vi "Keithley 182 Reading Config.VI"(1 "User Relative Value":dbl min=-30.3 max=30.3 format="%.9f", 2 "Reading Source":u16(ring) items=["Latest Reading from A/D", "One Reading from buffer", "All Readings in buffer", "Maximum Value in buffer", "Mimimum Value in buffer"], 4 "error in":T1, 5 "Analog Output Relative":u16(ring) items=["Disable Reading Relative", "Enable Reading Relative using current reading", "Enable Reading Relative using Value", "Enable Reading Relative, use present value"], 6 "Reading Format":u16(ring), 7 "VISA resource name":refnum<visa-resource-name>) -> (0 "error out":T1, 3 "VISA resource name out":refnum<visa-resource-name>)   [LabVIEW 2015]
doc: "This VI allows you to configure the 182 Reading source, format, and reading relative.\nOptions:\n\nReading Source\n0 = Latest Reading from A/D converter\n1 = One reading from buffer\n2 = All readings in buffer\n3 = Maximum value in buffer\n4 = Minimum value in buffer\n\nReading Format\n0 = Reading Only\n1 = Reading with prefix\n2 = Reading with buffer location\n3 = Reading with buffer location and prefix\n4 = Reading with time stamp\n5 = Reading with time stamp and prefix\n6 = Reading with time stamp and location\n7 = Reading with time stamp, location, and prefix\n\nReading Relative\n0 = Disable reading relative\n1 = Enable reading relative using next reading\n2 = Enable reading relative using value\n3 = Enable reading relative, using present value.\n\nReading relative value range => +/-1E-9 to +/-30.3"
panel:
  in  "?":string="Reading Relative Functions"
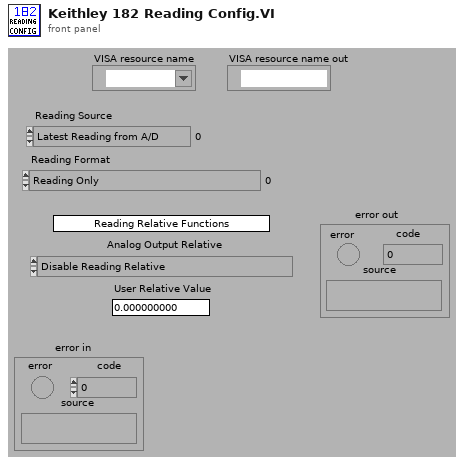
[diagram p1: front panel]
types:
  T1 = cluster{"error":bool, "code":i32, "source":string}
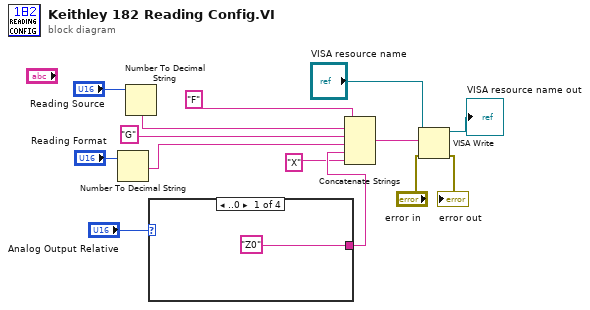
[diagram p0: block diagram]
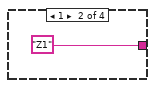
[diagram p2: hidden frame]
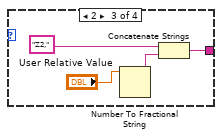
[diagram p3: hidden frame]
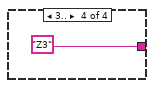
[diagram p4: hidden frame]
diagram:
  n1 = Number To Decimal String(number="Reading Format") -> (decimal integer string=w9:string)  [unwired: 1 out]
  n2 = Number To Decimal String(number="Reading Source") -> (decimal integer string=w13:string)  [unwired: 1 out]
  n3 = case shown="..0" "Analog Output Relative" {
    tunnel: ["Z0" "Z1" w19 "Z3"] -> w7
    frame ..0 {
    }
    frame 1 {
    }
    frame 2 {
      n4 = Number To Fractional String(number="User Relative Value") -> (F-format string=w18:string)  [unwired: 3 out]
      n5 = Concatenate Strings("Z2,", w18) -> (w19:string)
    }
    frame 3.. {
    }
  }
  n6 = Concatenate Strings("F", w13, "G", w9, w7, "X") -> (w5:string)
  n7 = VISA Write(VISA resource name="VISA resource name", write buffer=w5, error in (no error)="error in") -> (VISA resource name out=→"VISA resource name out":refnum<visa-resource-name>, error out=→"error out":errorcluster)  [unwired: 1 out]
